vi "Cargo Index Shoot.vi"() -> ()   [LabVIEW 2020]
uses:
  Team Code/Robot Global Data.vi
panel:
  in  "ShootDummy":bool
  out "LoopTime (ms)":u32
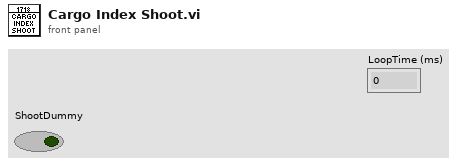
[diagram p1: front panel]
types:
  T1 = typedef "Trajectory_Library.lvlib/SWERVE_DRIVE_ODOMETRY.ctl" = cluster{"POSE":T2, "GyroOffset":T4, "PreviousAngle":T4, "PrevTime":dbl}
  T2 = typedef "Trajectory_Library.lvlib/POSE2D.ctl" = cluster{"TRANSLATION":T3, "ROTATION":T4}
  T3 = typedef "Trajectory_Library.lvlib/TRANSLATION2D.ctl" = cluster{"X":dbl, "Y":dbl}
  T4 = typedef "Trajectory_Library.lvlib/ROTATION2D.ctl" = cluster{"VALUE":dbl, "COS":dbl, "SIN":dbl}
  T5 = typedef "Cargo Sensors.ctl" = cluster{"ballPresent0":bool, "ballPresent1":bool, "ballPresent2":bool, "colorIsCorrect":bool, "ballPresent3":bool}
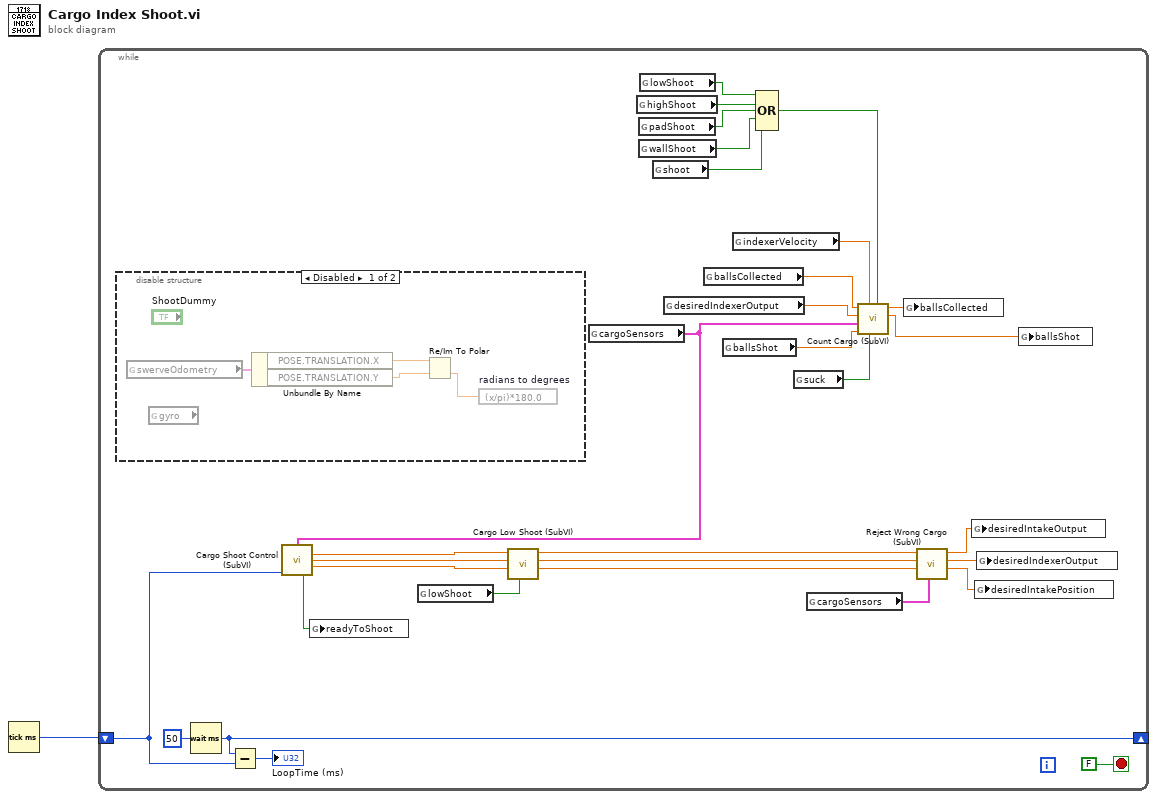
[diagram p0: block diagram]
diagram:
  n1 = Tick Count (ms)() -> (millisecond timer value=w1:u32)
  n2 = while {
    shift-right: [w26] -> _
    shift-left: w1 -> [w24]
    stop <- FALSE stop-if-true
    n3 = disable-structure shown="Disabled" {
      frame Disabled {
        n4 = global read "Robot Global Data.vi" "swerveOdometry"() -> (w36:T1)
        n5 = global read "Robot Global Data.vi" "gyro"() -> ()  [unwired: 1 out]
        n6 = Unbundle By Name(w36) -> ("POSE.TRANSLATION.X"=w35:dbl, "POSE.TRANSLATION.Y"=w34:dbl)
        n7 = Re/Im To Polar(2:w34, 3:w35) -> (0:w33:dbl)  [unwired: 1 out]
        n8 = expression code="(x/pi)*180.0" "radians to degrees"(w33) -> ()  [unwired: 1 out]
      }
      frame Enabled {
      }
    }
    n9 = Wait (ms)(milliseconds to wait=u32 50) -> (millisecond timer value=w26:u32)
    n10 = Subtract(x=w26, y=w24) -> (x-y=→"LoopTime (ms)":u32)
    n11 = global read "Robot Global Data.vi" "lowShoot"() -> (w12:bool)
    n12 = global read "Robot Global Data.vi" "cargoSensors"() -> (w25:T5)
    n13 = call "Cargo Shoot Control (SubVI).vi"("cargoSensors"=w25, "millisecond timer value"=w24) -> ("desiredIntakeOutput"=w18:dbl, "desiredIndexerOutput"=w19:dbl, "desiredIntakePosition"=w20:dbl, "readyToShoot"=w4:bool)  [unwired: 9 in, 1 out]
    n14 = global write "Robot Global Data.vi" "readyToShoot"(w4) -> ()
    n15 = call "Cargo Low Shoot (SubVI).vi"("lowShoot"=w12, "desiredIntakePosition"=w20, "desiredIndexerOutput"=w19, "desiredIntakeOutput"=w18) -> ("desiredIntakePosition"=w15:dbl, "desiredIndexerOutput"=w16:dbl, "desiredIntakeOutput"=w17:dbl)  [unwired: 5 in]
    n16 = global read "Robot Global Data.vi" "highShoot"() -> (w10:bool)
    n17 = global read "Robot Global Data.vi" "padShoot"() -> (w9:bool)
    n18 = global read "Robot Global Data.vi" "wallShoot"() -> (w8:bool)
    n19 = global read "Robot Global Data.vi" "lowShoot"() -> (w11:bool)
    n20 = global read "Robot Global Data.vi" "shoot"() -> (w7:bool)
    n21 = global read "Robot Global Data.vi" "desiredIndexerOutput"() -> (w3:dbl)
    n22 = global read "Robot Global Data.vi" "ballsCollected"() -> (w22:dbl)
    n23 = global read "Robot Global Data.vi" "ballsShot"() -> (w14:dbl)
    n24 = global read "Robot Global Data.vi" "indexerVelocity"() -> (w6:dbl)
    n25 = Compound Arithmetic op=OR(w11, w10, w9, w8, w7) -> (w5:bool)
    n26 = global read "Robot Global Data.vi" "suck"() -> (w2:bool)
    n27 = global read "Robot Global Data.vi" "cargoSensors"() -> (w31:T5)
    n28 = call "Count Cargo (SubVI).vi"("shooting"=w5, "sucking"=w2, "indexerVelocity"=w6, "ballsShotIn"=w14, "cargoSensors"=w25, "indexerDesired"=w3, "ballsCollectedIn"=w22) -> ("ballsShot"=w13:dbl, "ballsCollected"=w21:dbl)  [unwired: 3 in]
    n29 = global write "Robot Global Data.vi" "ballsCollected"(w21) -> ()
    n30 = call "Reject Wrong Cargo (SubVI).vi"("cargoSensors"=w31, "desiredIntakePosition"=w15, "desiredIndexerOutput"=w16, "desiredIntakeOutput"=w17) -> ("desiredIntakePosition"=w23:dbl, "desiredIndexerOutput"=w29:dbl, "desiredIntakeOutput"=w30:dbl)  [unwired: 5 in]
    n31 = global write "Robot Global Data.vi" "desiredIntakeOutput"(w30) -> ()
    n32 = global write "Robot Global Data.vi" "desiredIntakePosition"(w23) -> ()
    n33 = global write "Robot Global Data.vi" "desiredIndexerOutput"(w29) -> ()
    n34 = global write "Robot Global Data.vi" "ballsShot"(w13) -> ()
  }
